vi "Tosca-Trace-Open Log File.vi"(0 "Filestem":string, 11 "error in (no error)":errorcluster) -> (4 "refnum out":refnum<file>, 15 "error out":errorcluster)   [LabVIEW 2020]
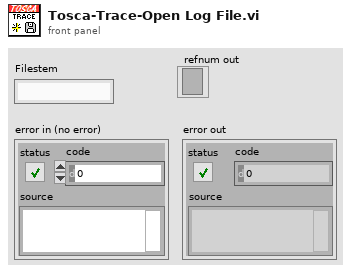
[diagram p1: front panel]
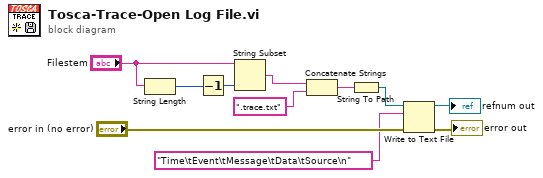
[diagram p0: block diagram]
diagram:
  n1 = String Length(string="Filestem") -> (length=w2:i32)
  n2 = Decrement(x=w2) -> (x-1=w3:i32)
  n3 = String Subset(string="Filestem", length (rest)=w3) -> (substring=w1:string)  [unwired: 1 in]
  n4 = Concatenate Strings(w1, ".trace.txt" ("string")) -> (w8:string)
  n5 = String To Path(string=w8) -> (path=w10:path)
  n6 = Write to Text File(file (use dialog)=w10, text="Time\tEvent\tMessage\tData\tSource\n", error in="error in (no error)") -> (refnum out=→"refnum out":refnum<file>, error out=→"error out":errorcluster)  [unwired: 1 in, 1 out]
